vi "Convert Array to Hex String.vi"(7 "Hex Array":u8[](array[numeric]) format="%.0x") -> (8 "String Message":string)   [LabVIEW 2016]
uses:
  <vilib>/Utility/error.llb/whitespace.ctl
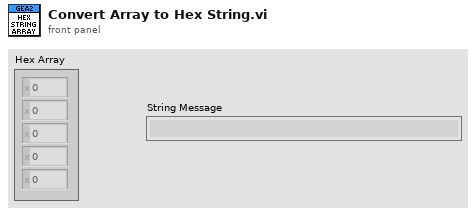
[diagram p1: front panel]
types:
  T1 = typedef "whitespace.ctl" = u16
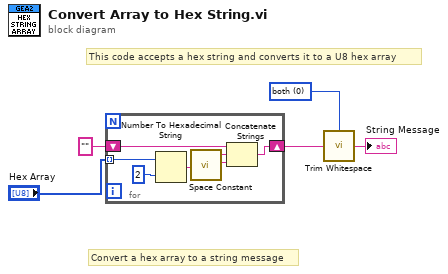
[diagram p0: block diagram]
diagram:
  w5 = T1 0 items=["both", "start of string", "end of string"] ("location (both)")
  # "Convert a hex array to a string message"
  # "This code accepts a hex string and converts it to a U8 hex array"
  n1 = for {
    tunnel: "Hex Array" -> [w11] mode=indexing
    shift-right: [w6] -> w3
    shift-left: "" -> [w9]
    n2 = Number To Hexadecimal String(1:i16 2 ("width (-)"), 2:w11) -> (0:w8:string)
    n3 = call <vilib>:"Space Constant.vi"() -> ("String"=w7:string)
    n4 = Concatenate Strings(w9, w8, w7) -> (w6:string)
  }
  n5 = call <vilib>:"Trim Whitespace.vi"("string"=w3, "location (both)"=w5) -> ("trimmed string"=→"String Message":string)
